vi "interpolate values.vi"(8 "error in (no error)":errorcluster, 9 "sample sage position":dbl[](array[numeric]) format="%_6g", 10 "focus position":dbl[](array[numeric]) format="%_6g", 11 "Autofocus in":refnum<class "Autofocus.lvclass">) -> (0 "error out":errorcluster, 2 "yi":dbl[](array[numeric]) format="%_6g", 3 "Autofocus out":refnum<class "Autofocus.lvclass">)   [LabVIEW 2012, in "Autofocus.lvclass"]
uses:
  Autofocus.lvclass
  Autofocus.lvclass/Autofocus.ctl
  <vilib>/gmath/NI_Gmath.lvlib
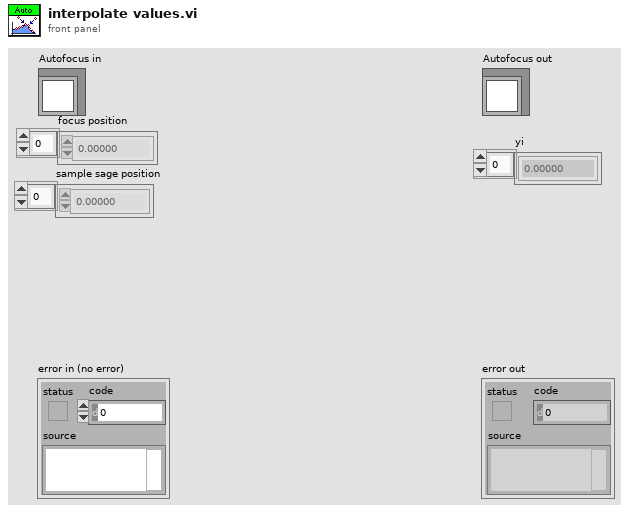
[diagram p1: front panel]
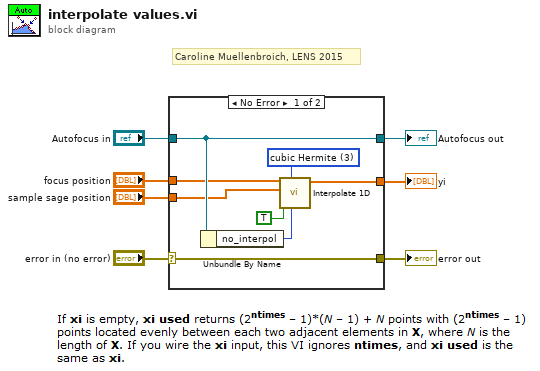
[diagram p0: block diagram]
diagram:
  # "Caroline Muellenbroich, LENS 2015"
  n1 = case shown="No Error" "error in (no error)" {
    selector: "error in (no error)" -> [w15 w17]
    tunnel: [w15 w17] -> w6
    tunnel: [w12 w16] -> w4
    tunnel: "Autofocus in" -> [w12 w16]
    tunnel: "focus position" -> [w10 _]
    tunnel: "sample sage position" -> [w9 _]
    tunnel: [w8 _] -> w1
    frame No Error {
      w13 = 3 items=["nearest", "linear", "spline", "cubic Hermite", "Lagrange"] ("method")
      n2 = Unbundle By Name(w12) -> ("no_interpol"=w11:i32)
      n3 = call <vilib>:"Interpolate 1D.vi"("ntimes"=w11, "method"=w13, "X is monotonic"=TRUE, "X"=w9, "Y"=w10) -> ("yi"=w8:dbl[])  [unwired: 4 in, 2 out]
    }
    frame Error {
    }
  }
  "error out" <- w6
  "Autofocus out" <- w4
  "yi" <- w1
